vi "G Byte Stream Writer.vi"(8 "error in (no error)":errorcluster, 10 "Value":variant, 11 "TwinCAT ADS in":refnum<class "TwinCAT ADS.lvclass">) -> (0 "error out":errorcluster, 1 "Byte Stream":u8[](array[numeric]), 3 "TwinCAT ADS out":refnum<class "TwinCAT ADS.lvclass">)   [LabVIEW 2018, in "TwinCAT ADS.lvclass"]
uses:
  TwinCAT ADS.lvclass
  <vilib>/Utility/Data Type/NI_Data Type.lvlib
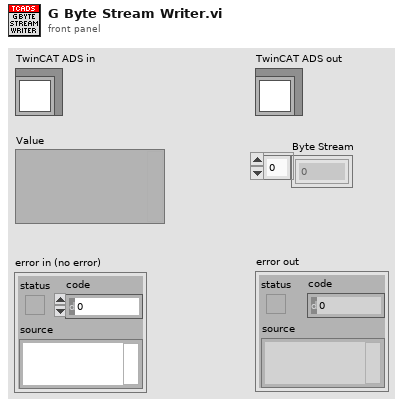
[diagram p1: front panel]
types:
  T1 = typedef "NI_Data Type.lvlib/Data Type.ctl" = enum8{"Invalid Type", "Void", "I8", "I16", "I32", "I64", "U8", "U16", "U32", "U64", "Single Float", "Double Float", "Extended Float", "Single Complex", "Double Complex", "Extended Complex", "Enum U8", "Enum U16", "Enum U32", "Enum U64", "Single Float With Unit", "Double Float With Unit", "Extended Float With Unit", "Single Complex with Unit", "Double Complex with Unit", "Extended Complex with Unit", "Boolean", "String", "Path", "Picture", "Tag", "Array", "Cluster", "Variant", "LV Variant", "Waveform", "Timestamp", "Digital Waveform", "Digital Data", "ExpressData", "Refnum", "External Data", "VI", "Poly VI", "LabVIEW Class Instance", "Fixed Point"}
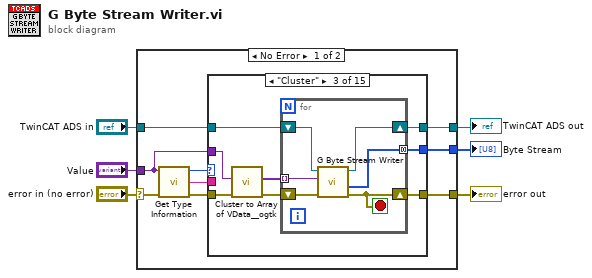
[diagram p0: block diagram]
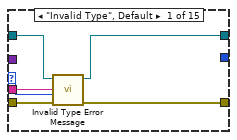
[diagram p2: hidden frame]
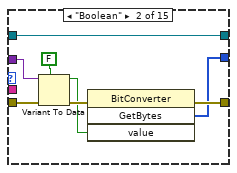
[diagram p3: hidden frame]
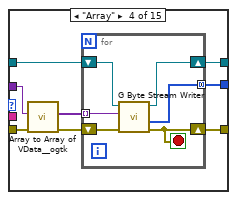
[diagram p4: hidden frame]
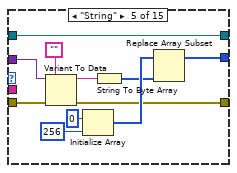
[diagram p5: hidden frame]
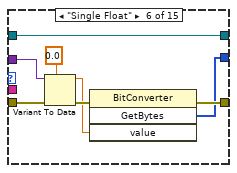
[diagram p6: hidden frame]
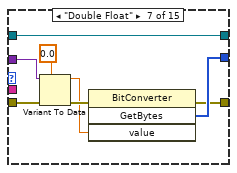
[diagram p7: hidden frame]
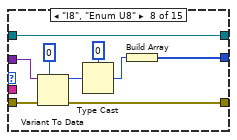
[diagram p8: hidden frame]
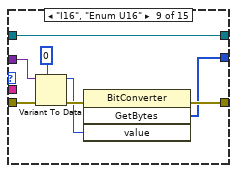
[diagram p9: hidden frame]
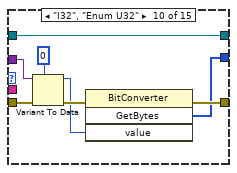
[diagram p10: hidden frame]
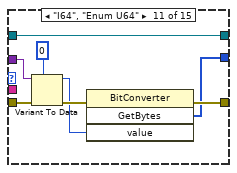
[diagram p11: hidden frame]
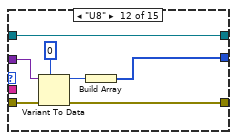
[diagram p12: hidden frame]
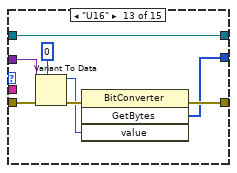
[diagram p13: hidden frame]
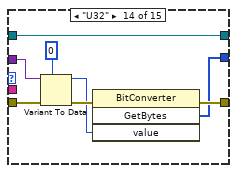
[diagram p14: hidden frame]
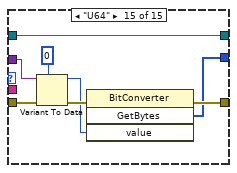
[diagram p15: hidden frame]
diagram:
  n1 = case shown="No Error" "error in (no error)" {
    selector: "error in (no error)" -> [w15 w150]
    tunnel: [w7 w150] -> w5
    tunnel: [w8 w149] -> w3
    tunnel: "TwinCAT ADS in" -> [w13 w149]
    tunnel: "Value" -> [w10 _]
    tunnel: [w9 _] -> w1
    frame No Error {
      n2 = call <vilib>:"Get Type Information.vi"("error in (no error)"=w15, "Variant"=w10) -> ("error out"=w14:errorcluster, "Name"=w11:string, "Type"=w12:T1)  [unwired: 5 in, 2 out]
      n3 = case shown="\"Cluster\"" w12 {
        selector: w12 -> [w19 _ _ _ _ _ _ _ _ _ _ _ _ _ _]
        tunnel: w10 -> [_ w29 w36 w47 w68 w76 w84 w93 w101 w109 w117 w124 w132 w140 w148]
        tunnel: [w20 w23 w31 w49 w60 w71 w77 w87 w95 w103 w111 w119 w126 w135 w143] -> w7
        tunnel: w14 -> [w21 w26 w37 w46 w67 w74 w82 w91 w99 w106 w115 w121 w131 w138 w145]
        tunnel: w13 -> [w17 w28 w33 w51 w66 w75 w83 w92 w100 w107 w116 w122 w128 w139 w146]
        tunnel: [w16 w28 w32 w50 w66 w75 w83 w92 w100 w107 w116 w122 w128 w139 w146] -> w8
        tunnel: [_ w22 w30 w48 w59 w70 w79 w85 w94 w102 w110 w118 w125 w134 w142] -> w9
        tunnel: w11 -> [w18 _ _ _ _ _ _ _ _ _ _ _ _ _ _]
        frame "Invalid Type", Default {
          n4 = call "Invalid Type Error Message.vi"("error in (no error)"=w21, "Type"=w19, "Name"=w18, "TwinCAT ADS in"=w17) -> ("error out"=w20:errorcluster, "TwinCAT ADS out"=w16:refnum<class "TwinCAT ADS.lvclass">)  [unwired: 6 in]
        }
        frame "Boolean" {
          n5 = Variant To Data(error in=w26, type=FALSE, Variant=w29) -> (data=w24:bool, error out=w25:errorcluster)
          n6 = invoke class="BitConverter" method="GetBytes"(error in=w25, "value"=w24) -> (error out=w23:errorcluster, "GetBytes"=w22:u8[])  [unwired: 2 in, 2 out]
        }
        frame "Cluster" {
          n7 = call <userlib>:"Cluster to Array of VData__ogtk.vi"("error in (no error)"=w37, "Cluster"=w36) -> ("error out"=w35:errorcluster, "Array of VData"=w34:variant[])  [unwired: 8 in]
          n8 = for {
            tunnel: w34 -> [w42] mode=indexing
            shift-right: [w38] -> w31
            shift-left: w35 -> [w43]
            shift-right: [w40] -> w32
            shift-left: w33 -> [w41]
            tunnel: [w39] -> w30 mode=concatenating
            stop <- w38 stop-if-true
            n9 = call-dynamic "G Byte Stream Writer.vi"("error in (no error)"=w43, "Value"=w42, "TwinCAT ADS in"=w41) -> ("error out"=w38:errorcluster, "Byte Stream"=w39:u8[], "TwinCAT ADS out"=w40:refnum<class "TwinCAT ADS.lvclass">)  [unwired: 6 in]
          }
        }
        frame "Array" {
          n10 = call <userlib>:"Array to Array of VData__ogtk.vi"("error in (no error)"=w46, "MultiD Array"=w47) -> ("error out"=w45:errorcluster, "1D Array of Variants"=w44:variant[])  [unwired: 8 in]
          n11 = for {
            tunnel: w44 -> [w56] mode=indexing
            shift-right: [w52] -> w49
            shift-left: w45 -> [w57]
            shift-right: [w54] -> w50
            shift-left: w51 -> [w55]
            tunnel: [w53] -> w48 mode=concatenating
            stop <- w52 stop-if-true
            n12 = call-dynamic "G Byte Stream Writer.vi"("error in (no error)"=w57, "Value"=w56, "TwinCAT ADS in"=w55) -> ("error out"=w52:errorcluster, "Byte Stream"=w53:u8[], "TwinCAT ADS out"=w54:refnum<class "TwinCAT ADS.lvclass">)  [unwired: 6 in]
          }
        }
        frame "String" {
          n13 = Variant To Data(error in=w67, type="", Variant=w68) -> (data=w65:string, error out=w60:errorcluster)
          n14 = Initialize Array(u8 0, 256 ("length")) -> (w62:u8[])
          n15 = String To Byte Array(string=w65) -> (unsigned byte array=w61:u8[])
          n16 = Replace Array Subset(array=w62, new element=w61) -> (w59:u8[])  [unwired: 1 in]
        }
        frame "Single Float" {
          n17 = Variant To Data(error in=w74, type=sgl 0.0 ("value"), Variant=w76) -> (data=w72:sgl, error out=w73:errorcluster)
          n18 = invoke class="BitConverter" method="GetBytes"(error in=w73, "value"=w72) -> (error out=w71:errorcluster, "GetBytes"=w70:u8[])  [unwired: 2 in, 2 out]
        }
        frame "Double Float" {
          n19 = Variant To Data(error in=w82, type=0.0 ("value"), Variant=w84) -> (data=w80:dbl, error out=w81:errorcluster)
          n20 = invoke class="BitConverter" method="GetBytes"(error in=w81, "value"=w80) -> (error out=w77:errorcluster, "GetBytes"=w79:u8[])  [unwired: 2 in, 2 out]
        }
        frame "I8", "Enum U8" {
          n21 = Variant To Data(error in=w91, type=i8 0 ("value"), Variant=w93) -> (data=w89:i8, error out=w87:errorcluster)
          n22 = Type Cast(type=u8 0, x=w89) -> (*(type *) &x=w86:u8)
          n23 = Build Array(w86) -> (w85:u8[])
        }
        frame "I16", "Enum U16" {
          n24 = Variant To Data(error in=w99, type=i16 0 ("value"), Variant=w101) -> (data=w96:i16, error out=w97:errorcluster)
          n25 = invoke class="BitConverter" method="GetBytes"(error in=w97, "value"=w96) -> (error out=w95:errorcluster, "GetBytes"=w94:u8[])  [unwired: 2 in, 2 out]
        }
        frame "I32", "Enum U32" {
          n26 = Variant To Data(error in=w106, type=0 ("value"), Variant=w109) -> (data=w104:i32, error out=w105:errorcluster)
          n27 = invoke class="BitConverter" method="GetBytes"(error in=w105, "value"=w104) -> (error out=w103:errorcluster, "GetBytes"=w102:u8[])  [unwired: 2 in, 2 out]
        }
        frame "I64", "Enum U64" {
          n28 = Variant To Data(error in=w115, type=i64 0 ("value"), Variant=w117) -> (data=w112:i64, error out=w113:errorcluster)
          n29 = invoke class="BitConverter" method="GetBytes"(error in=w113, "value"=w112) -> (error out=w111:errorcluster, "GetBytes"=w110:u8[])  [unwired: 2 in, 2 out]
        }
        frame "U8" {
          n30 = Variant To Data(error in=w121, type=u8 0 ("value"), Variant=w124) -> (data=w120:u8, error out=w119:errorcluster)
          n31 = Build Array(w120) -> (w118:u8[])
        }
        frame "U16" {
          n32 = Variant To Data(error in=w131, type=u16 0 ("value"), Variant=w132) -> (data=w129:u16, error out=w130:errorcluster)
          n33 = invoke class="BitConverter" method="GetBytes"(error in=w130, "value"=w129) -> (error out=w126:errorcluster, "GetBytes"=w125:u8[])  [unwired: 2 in, 2 out]
        }
        frame "U32" {
          n34 = Variant To Data(error in=w138, type=u32 0 ("value"), Variant=w140) -> (data=w133:u32, error out=w136:errorcluster)
          n35 = invoke class="BitConverter" method="GetBytes"(error in=w136, "value"=w133) -> (error out=w135:errorcluster, "GetBytes"=w134:u8[])  [unwired: 2 in, 2 out]
        }
        frame "U64" {
          n36 = Variant To Data(error in=w145, type=u64 0 ("value"), Variant=w148) -> (data=w141:u64, error out=w144:errorcluster)
          n37 = invoke class="BitConverter" method="GetBytes"(error in=w144, "value"=w141) -> (error out=w143:errorcluster, "GetBytes"=w142:u8[])  [unwired: 2 in, 2 out]
        }
      }
    }
    frame Error {
    }
  }
  "error out" <- w5
  "TwinCAT ADS out" <- w3
  "Byte Stream" <- w1
